vi "ShootV1.vi"(11 "Butons":bool[](array[boolean])) -> ()   [LabVIEW 2015]
uses:
  Utilities/ShootControl.ctl
  <vilib>/Rock Robotics/WPI/Solenoid/WPI_SolenoidValue.ctl
  Utilities/GlobalVisionVars.vi
  Utilities/VisionGlobals.vi
  Utilities/GeneralGlobals.vi
  Utilities/MotorPositionGlobals.vi
  <vilib>/Rock Robotics/WPI/Solenoid/WPI_SolenoidSetEnum.vi
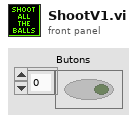
[diagram p1: front panel]
types:
  T1 = typedef "ShootControl.ctl" = enum16{"WaitingForInput", "Shoot", "Reload", "Release"}
  T2 = typedef "WPI_SolenoidDevRef.ctl" = cluster{"DevStatus":errorcluster, "Pneumatics Control Module":u8, "Forward Solenoid Channel":T3, "Reverse Solenoid Channel":T3}
  T3 = typedef "WPI_SolenoidChannel.ctl" = enum8{"Solenoid 0", "Solenoid 1", "Solenoid 2", "Solenoid 3", "Solenoid 4", "Solenoid 5", "Solenoid 6", "Solenoid 7", "Invalid"}
  T4 = typedef "WPI_SolenoidValue.ctl" = enum16{"Off", "On", "Forward", "Reverse"}
  T5 = typedef "WPI_MotorControlDeviceRef.ctl" = cluster{"DeviceStatus":errorcluster, "Type":T6, "PWM":cluster{"PWM Channel":T7, "DeadBand":T8}, "CAN":cluster{"Device Number":u8, "Control Mode":T9, "Semaphore":T10, "Max Vout":dbl, "TalonSRX Control Mode":T11}, "Invert":bool}
  T6 = typedef "WPI_MotorControlType.ctl" = enum16{"PWM", "CAN", "CANTalonSRX"}
  T7 = typedef "FPGA_DIOPWMChannel.ctl" = enum8{"PWM 0", "PWM 1", "PWM 2", "PWM 3", "PWM 4", "PWM 5", "PWM 6", "PWM 7", "PWM 8", "PWM 9", "PWM MXP 0", "PWM MXP 1", "PWM MXP 2", "PWM MXP 3", "PWM MXP 4", "PWM MXP 5", "PWM MXP 6", "PWM MXP 7", "PWM MXP 8", "PWM MXP 9", "Invalid"}
  T8 = typedef "WPI_PWMDeadband.ctl" = cluster{"Name":string, "maxPositivePwm":i32, "minPositivePwm":i32, "centerPwm":i32, "maxNegativePwm":i32, "minNegativePwm":i32, "angularRange":u16}
  T9 = typedef "WPI_CANJaguar_ControlMode.ctl" = enum8{"Percent VBus", "Current", "Speed", "Position", "Voltage"}
  T10 = typedef "Semaphore RefNum" = refnum<k1>
  T11 = typedef "WPI_CANTalonSRX_APIControlMode.ctl" = enum8{"Percent VBus", "Speed", "Position", "Slave", "Unchanged / Invalid", "Voltage Compensation", "Current", "Motion Profile"}
  T12 = typedef "WPI_CANTalonSRX_GlobalStatus.ctl" = cluster{"Applied Throttle":dbl, "Module Enabled":bool, "CAN Error":errorcluster, "Closed Loop Error":dbl, "Forward Limit Switch Closed":bool, "Reverse Limit Switch Closed":bool, "Sensor Position":dbl, "Sensor Velocity":dbl, "Current":dbl, "Sticky Fault - Over Temp":bool, "Sticky Fault - Under Voltage":bool, "Sticky Fault - Forward Limit":bool, "Sticky Fault - Reverse Limit":bool, "Sticky Fault - Forward Soft Limit":bool, "Sticky Fault - Reverse Soft Limit":bool, "Brake is Enabled":bool, "Encoder Position":dbl, "Encoder Velocity":dbl, "Encoder Index Count":dbl, "Encoder A Pin State":bool, "Encoder B Pin State":bool, "Encoder Index Pin State":bool, "Analog In":dbl, "Analog In Velocity":dbl, "Temperature (C)":dbl, "Battery Voltage":dbl, "Control 5 Is Supported":bool, "Current Profile Slot Select":dbl, "Pos Div 8":bool, "Vel Div 4":bool, "Pulse Width Position":i32, "Pulse Width Velocity":i32, "Pulse Width Rise To Rise (us)":i32, "Pulse Width Rise To Fall (us)":i32, "Mot Prof Active Is Under Run":bool, "Mot Prof Active Has Under Run":bool, "Mot Prof Active Is Last":bool, "Mot Prof Active Velocity Only":bool, "Mot Prof Active Is Valid":bool, "Mot Prof Buffer Is Full":bool, "Mot Prof Active Profile Slot Select":i32, "Mot Prof NextID":i32, "Mot Prof Count":i32, "Mot Prof Active Velocity":dbl, "Mot Prof Active Position":dbl, "Mot Prof Output Enable":i32}
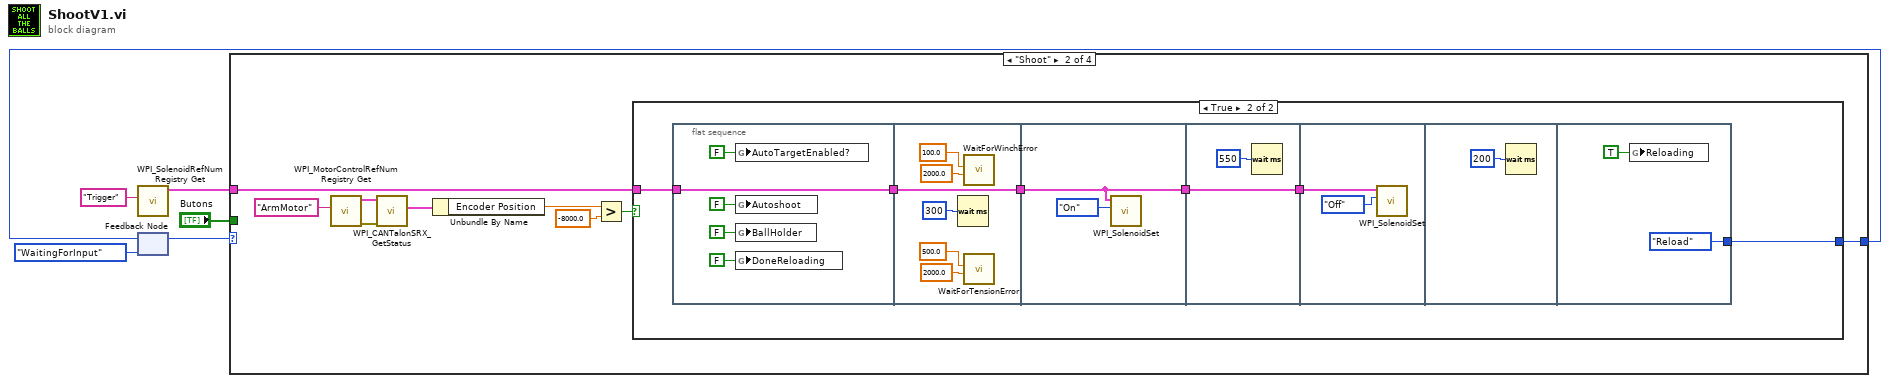
[diagram p0: block diagram]
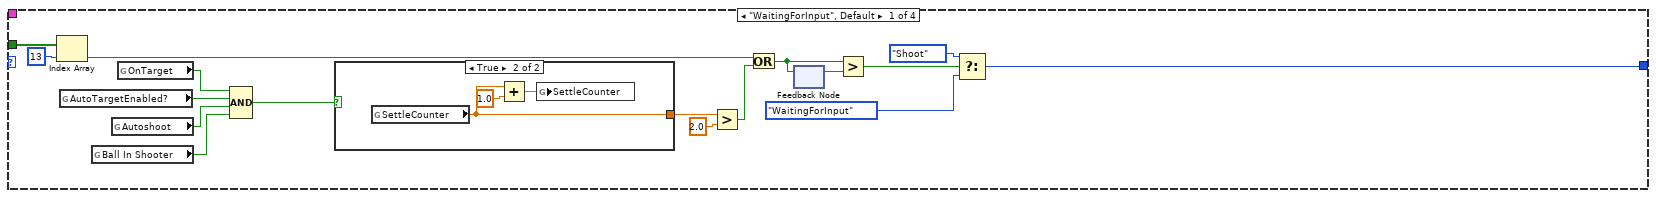
[diagram p2: hidden frame]
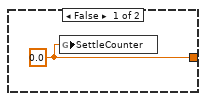
[diagram p3: hidden frame]
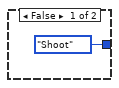
[diagram p4: hidden frame]
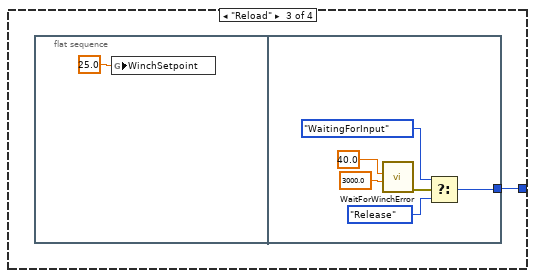
[diagram p5: hidden frame]
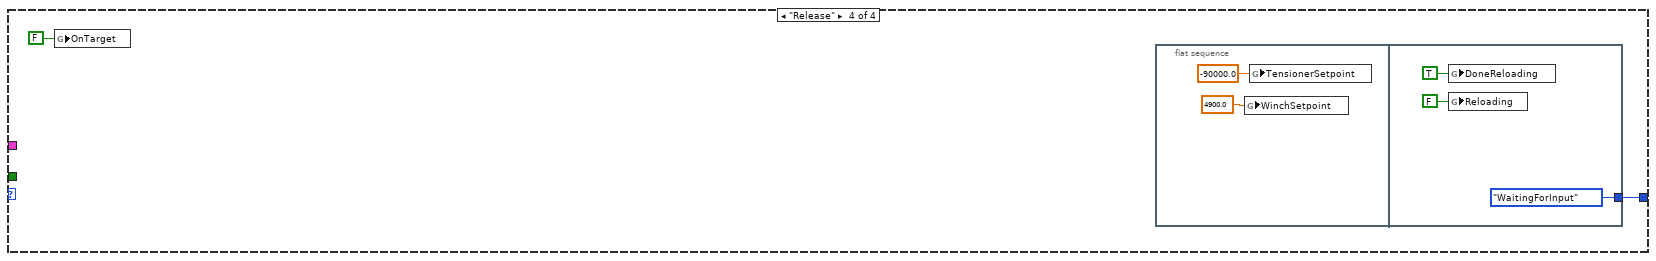
[diagram p6: hidden frame]
diagram:
  n1 = call <vilib>:"WPI_SolenoidRefNum Registry Get.vi"("refnum name"="Trigger") -> ("SolenoidDevRef"=w1:T2)  [unwired: 9 in, 1 out]
  n2 = feedback #1(ShootControl."WaitingForInput" ("Enum")) -> (w6:T1)
  n3 = case shown="\"Shoot\"" w6 {
    tunnel: "Butons" -> [w23 _ _ _]
    tunnel: [w17 w35 w64 w73] -> w3
    tunnel: w1 -> [_ w36 _ _]
    frame "WaitingForInput", Default {
      n4 = Index Array(array=w23, index=13) -> (element=w15:bool)
      n5 = global read "VisionGlobals.vi" "AutoTargetEnabled?"() -> (w10:bool)
      n6 = global read "GeneralGlobals.vi" "Ball In Shooter"() -> (w7:bool)
      n7 = global read "VisionGlobals.vi" "Autoshoot"() -> (w11:bool)
      n8 = global read "GlobalVisionVars.vi" "OnTarget"() -> (w9:bool)
      n9 = Compound Arithmetic op=AND(w9, w10, w11, w7) -> (w8:bool)
      n10 = case shown="True" w8 {
        tunnel: [w24 w25] -> w13
        frame False {
          w24 = 0.0 ("SettleCounter")
          n11 = global write "GlobalVisionVars.vi" "SettleCounter"(w24) -> ()
        }
        frame True {
          n12 = global read "GlobalVisionVars.vi" "SettleCounter"() -> (w25:dbl)
          n13 = Add(x=w25, y=1.0) -> (x+y=w26:dbl)
          n14 = global write "GlobalVisionVars.vi" "SettleCounter"(w26) -> ()
        }
      }
      n15 = Greater?(x=w13, y=2.0) -> (0:w12:bool)
      n16 = Or(x=w15, y=w12) -> (x .or. y?=w16:bool)
      n17 = feedback-in #2(w16) -> ()
      n18 = feedback #2() -> (w21:bool)  [unwired: 1 in]
      n19 = Greater?(x=w16, y=w21) -> (0:w20:bool)
      n20 = Select(t=ShootControl."Shoot" ("Enum"), s=w20, f=ShootControl."WaitingForInput" ("Enum")) -> (s? t:f=w17:T1)
    }
    frame "Shoot" {
      n21 = call <vilib>:"WPI_MotorControlRefNum Registry Get.vi"("refnum name"="ArmMotor") -> ("error out"=w33:errorcluster, "MotorControlDevRef"=w32:T5)  [unwired: 9 in]
      n22 = call <vilib>:"WPI_CANTalonSRX_GetStatus.vi"("error in (no error)"=w33, "CAN Talon SRX Ref"=w32) -> ("Talon SRX Status"=w31:T12)  [unwired: 7 in, 2 out]
      n23 = Unbundle By Name(w31) -> ("Encoder Position"=w29:dbl)
      n24 = Greater?(x=w29, y=-8000.0) -> (0:w30:bool)
      n25 = case shown="True" w30 {
        tunnel: w36 -> [_ w39]
        tunnel: [ShootControl."Shoot" ("Enum") w38] -> w35
        frame False {
        }
        frame True {
          n26 = flat-sequence {
            tunnel: w39 -> [w48]
            tunnel: [w48] -> w43
            tunnel: w43 -> [w54]
            tunnel: [w54] -> w42
            tunnel: [w55] -> w41
            tunnel: w42 -> [w55]
            tunnel: w41 -> [w57]
            tunnel: [w57] -> w40
            tunnel: w40 -> [w59]
            tunnel: [ShootControl."Reload" ("Enum")] -> w38
            frame #0 {
              n27 = global write "VisionGlobals.vi" "AutoTargetEnabled?"(FALSE ("AutoTargetEnabled?")) -> ()
              n28 = global write "VisionGlobals.vi" "Autoshoot"(FALSE ("Autoshoot")) -> ()
              n29 = global write "MotorPositionGlobals.vi" "BallHolder"(FALSE ("BallHolder")) -> ()
              n30 = global write "GeneralGlobals.vi" "DoneReloading"(FALSE ("DoneReloading")) -> ()
            }
            frame #1 {
              n31 = Wait (ms)(milliseconds to wait=u32 300) -> ()  [unwired: 1 out]
              n32 = call "WaitForWinchError.vi"("Timeout (ms)"=2000.0, "AllowedError"=100.0) -> ()  [unwired: 9 in, 1 out]
              n33 = call "WaitForTensionError.vi"("Timeout (ms)"=2000.0, "AllowedError"=500.0) -> ()  [unwired: 9 in, 1 out]
            }
            frame #2 {
              n34 = call-poly <vilib>:"WPI_SolenoidSet.vi"("Value"=WPI_SolenoidValue."On", "SolenoidDevRef"=w55) -> ()  [unwired: 8 in, 2 out]
            }
            frame #3 {
              n35 = Wait (ms)(milliseconds to wait=u32 550) -> ()  [unwired: 1 out]
            }
            frame #4 {
              n36 = call-poly <vilib>:"WPI_SolenoidSet.vi"("Value"=WPI_SolenoidValue."Off", "SolenoidDevRef"=w59) -> ()  [unwired: 8 in, 2 out]
            }
            frame #5 {
              n37 = Wait (ms)(milliseconds to wait=u32 200) -> ()  [unwired: 1 out]
            }
            frame #6 {
              n38 = global write "GeneralGlobals.vi" "Reloading"(TRUE ("DoneReloading")) -> ()
            }
          }
        }
      }
    }
    frame "Reload" {
      n39 = flat-sequence {
        tunnel: [w67] -> w64
        frame #0 {
          n40 = global write "MotorPositionGlobals.vi" "WinchSetpoint"(25.0 ("WinchPosition")) -> ()
        }
        frame #1 {
          n41 = call "WaitForWinchError.vi"("Timeout (ms)"=3000.0, "AllowedError"=40.0) -> ("error out"=w69:errorcluster)  [unwired: 9 in]
          n42 = Select(t=ShootControl."WaitingForInput" ("Enum"), s=w69, f=ShootControl."Release" ("Enum")) -> (s? t:f=w67:T1)
        }
      }
    }
    frame "Release" {
      n43 = global write "GlobalVisionVars.vi" "OnTarget"(FALSE ("OnTarget")) -> ()
      n44 = flat-sequence {
        tunnel: [ShootControl."WaitingForInput" ("Enum")] -> w73
        frame #0 {
          n45 = global write "MotorPositionGlobals.vi" "WinchSetpoint"(4900.0 ("WinchSetpoint")) -> ()
          n46 = global write "MotorPositionGlobals.vi" "TensionerSetpoint"(-90000.0 ("TensionerSetpoint")) -> ()
        }
        frame #1 {
          n47 = global write "GeneralGlobals.vi" "DoneReloading"(TRUE ("DoneReloading")) -> ()
          n48 = global write "GeneralGlobals.vi" "Reloading"(FALSE ("DoneReloading")) -> ()
        }
      }
    }
  }
  n49 = feedback-in #1(w3) -> ()
